vi "MVP valve command and read.vi"(5 "error in":errorcluster, 6 "command\n(w/o pump # prefix)":string, 7 "Valve # (1=a, 2=b, ....  0 = no prefix)":u8, 8 "VISA resource name":refnum<visa-resource-name>="VALVE") -> (0 "error out":errorcluster, 1 "Output String":string, 3 "VISA resource name out":refnum<visa-resource-name>)   [LabVIEW 2015]
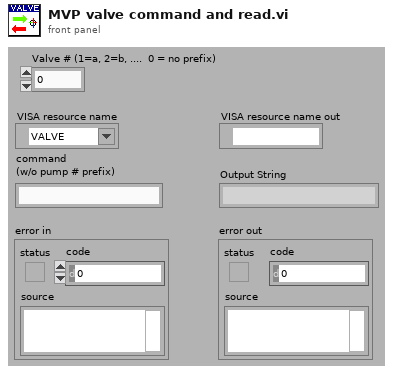
[diagram p1: front panel]
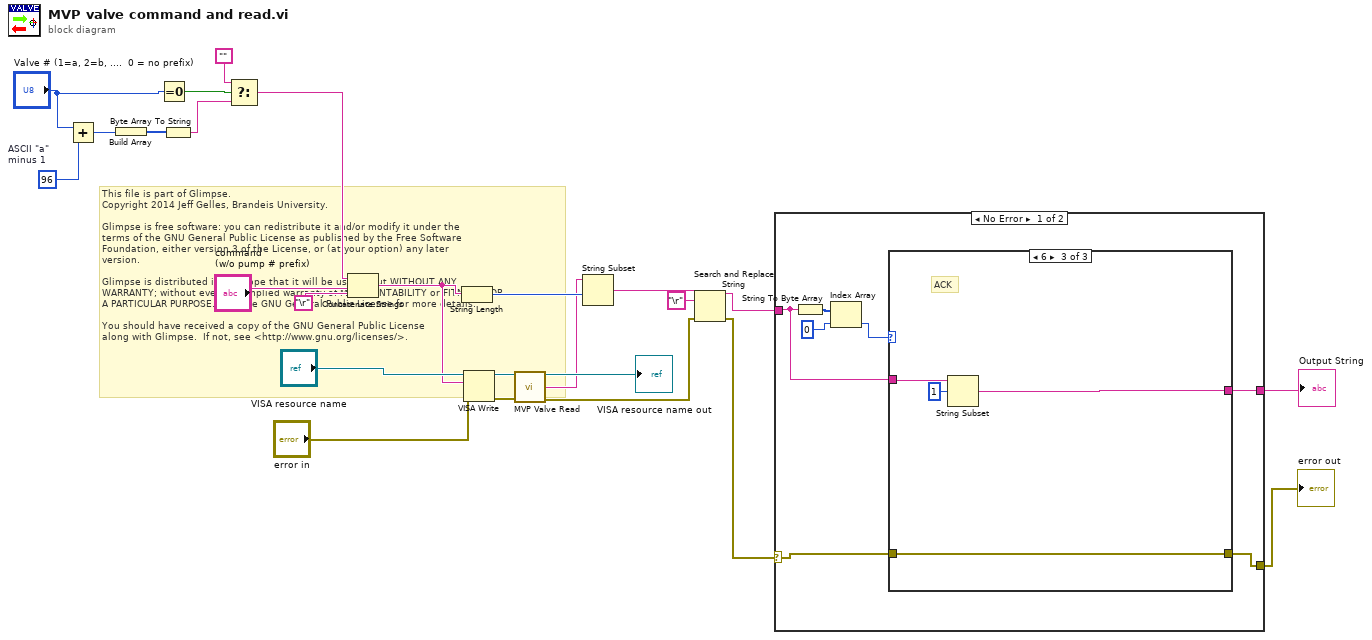
[diagram p0: block diagram]
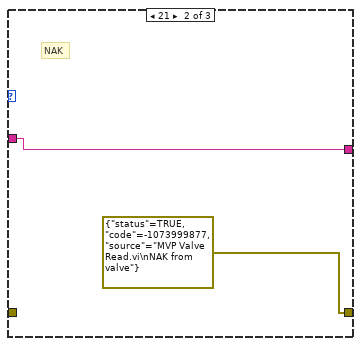
[diagram p3: hidden frame]
diagram:
  w8 = u8 96  # ASCII "a" minus 1
  # "This file is part of Glimpse. \nCopyright 2014 Jeff Gelles, Brandeis University.    \n\nGlimpse is free software: you can redistribute it and/or modify it under the \nterms of the GNU General Public License as published by the Free Software \nFoundation, either version 3 of the License, or (at your option) any later \nversion.\n\nGlimpse is distributed in the hope that it will be useful, but WITHOUT ANY \nWARRANTY; without even the implied warranty of MERCHANTABILITY or FITNESS FOR \nA PARTICULAR PURPOSE.  See the GNU General Public License for more details.\n\nYou should have received a copy of the GNU General Public License\nalong with Glimpse.  If not, see <http://www.gnu.org/licenses/>."
  n1 = Add(x="Valve # (1=a, 2=b, ....  0 = no prefix)", y=w8) -> (x+y=w7:u8)
  n2 = Build Array(w7) -> (w6:u8[])
  n3 = Equal To 0?(x="Valve # (1=a, 2=b, ....  0 = no prefix)") -> (x = 0?=w4:bool)
  n4 = Byte Array To String(unsigned byte array=w6) -> (string=w3:string)
  n5 = Select(t="", s=w4, f=w3) -> (s? t:f=w1:string)
  n6 = Concatenate Strings(w1, "command\n(w/o pump # prefix)", "\r") -> (w18:string)
  n7 = String Length(string=w18) -> (length=w17:i32)
  n8 = VISA Write(VISA resource name="VISA resource name", write buffer=w18, error in (no error)="error in") -> (VISA resource name out=w23:refnum<visa-resource-name>, error out=w22:errorcluster)  [unwired: 1 out]
  n9 = call "MVP Valve Read.vi"("VISA resource name"=w23, "error in (no error)"=w22) -> ("VISA resource name out"=→"VISA resource name out":refnum<visa-resource-name>, "Output String"=w16:string, "error out"=w13:errorcluster)  [unwired: 11 out]
  n10 = String Subset(string=w16, offset (0)=w17) -> (substring=w15:string)  [unwired: 1 out]
  n11 = Search and Replace String(input string=w15, search string="\r", error in=w13) -> (result string=w12:string, error out=w9:errorcluster)  [unwired: 7 out]
  n12 = case shown="No Error" w9 {
    selector: w9 -> [w27 w42]
    tunnel: w12 -> [w29 w41]
    tunnel: [w26 w42] -> w10
    tunnel: [w28 w41] -> w11
    frame No Error {
      n13 = String To Byte Array(string=w29) -> (unsigned byte array=w32:u8[])
      n14 = Index Array(array=w32, index=0 ("length (rest)")) -> (element=w30:u8)
      n15 = case shown="6" w30 {
        tunnel: w29 -> [w34 w35 w40]
        tunnel: [w34 w35 w38] -> w28
        tunnel: w27 -> [w33 _ w37]
        tunnel: [w33 errorcluster {"status"=TRUE, "code"=-1073999877, "source"="MVP Valve Read.vi\nNAK from valve"} ("t") w37] -> w26
        frame Default {
        }
        frame 21 {
          # "NAK"
        }
        frame 6 {
          # "ACK"
          n16 = String Subset(string=w40, offset (0)=1) -> (substring=w38:string)  [unwired: 1 out]
        }
      }
    }
    frame Error {
    }
  }
  "Output String" <- w11
  "error out" <- w10
